vi "Cluster Get All Control Names&Values.vi"(11 "xml string":string) -> (2 "value":string[](array[string]), 3 "name":string[](array[string]))   [LabVIEW 2020]
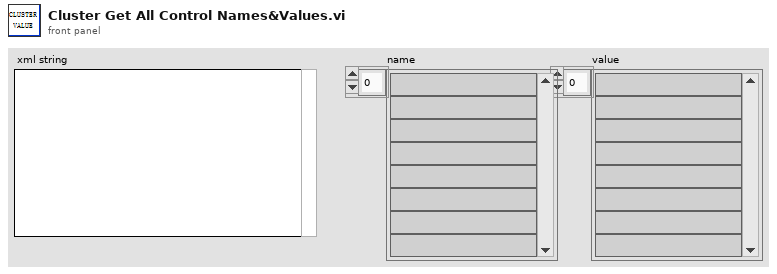
[diagram p1: front panel]
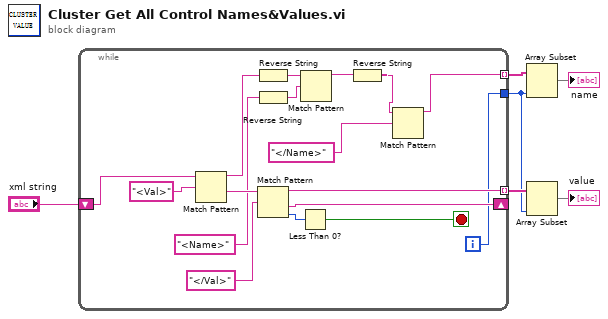
[diagram p0: block diagram]
diagram:
  n1 = while {
    tunnel: [w19] -> w2 mode=indexing
    shift-right: [w17] -> _
    shift-left: "xml string" -> [w23]
    tunnel: [w7] -> w5 mode=indexing
    tunnel: [w11] -> w1
    i -> [w11]
    stop <- w18 stop-if-true
    n2 = Match Pattern(string=w23, regular expression="<Val>" ("正则表达式")) -> (before substring=w15:string, after substring=w21:string)  [unwired: 1 in, 2 out]
    n3 = Reverse String(1:w15) -> (0:w14:string)
    n4 = Reverse String(1:"<Name>" ("正则表达式")) -> (0:w12:string)
    n5 = Match Pattern(string=w21, regular expression="</Val>" ("正则表达式")) -> (before substring=w19:string, after substring=w17:string, offset past match=w16:i32)  [unwired: 1 in, 1 out]
    n6 = Less Than 0?(x=w16) -> (x < 0?=w18:bool)
    n7 = Match Pattern(string=w14, regular expression=w12) -> (before substring=w10:string)  [unwired: 1 in, 3 out]
    n8 = Reverse String(1:w10) -> (0:w8:string)
    n9 = Match Pattern(string=w8, regular expression="</Name>" ("正则表达式")) -> (before substring=w7:string)  [unwired: 1 in, 3 out]
  }
  n10 = Array Subset(array=w5, length=w1) -> (→"name":string[])  [unwired: 1 in]
  n11 = Array Subset(array=w2, length=w1) -> (→"value":string[])  [unwired: 1 in]
